vi "Execute SQL Command (no data returned).vi"(4 "error in":errorcluster, 6 "SQL Command":string, 7 "Connection In":refnum<k7>) -> (0 "error out":errorcluster, 1 "records effected":i32, 3 "Connection Out":refnum<k7>)   [LabVIEW 2022 SP3, in "hse-db-ado.lvlib" / "ADO-DB-Driver.lvlib"]
doc: "Execute a SQL command without returning any data\n\n____\nHAMPEL SOFTWARE ENGINEERING v1.4.0 (2023-12-19 09:52)"
uses:
  ADO-DB-Driver.lvlib
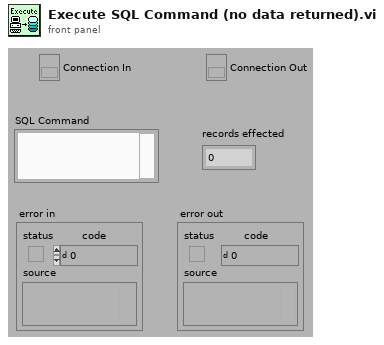
[diagram p1: front panel]
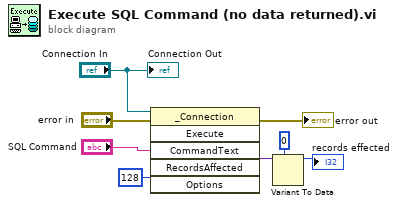
[diagram p0: block diagram]
diagram:
  n1 = invoke class="_Connection" method="Execute"(reference="Connection In", error in="error in", "CommandText"="SQL Command", "Options"=128) -> (error out=→"error out":errorcluster, "RecordsAffected"=w8:variant)  [unwired: 2 in, 4 out]
  n2 = Variant To Data(type=0, Variant=w8) -> (data=→"records effected":i32)  [unwired: 1 in, 1 out]
  "Connection Out" <- "Connection In"
